vi "_readEscapeSequence.vi"(8 "error in (no error)":errorcluster, 11 "tJSONParser in":refnum<class "tJSONParser.lvclass">) -> (0 "error out":errorcluster, 2 "String Out":string, 3 "tJSONParser out":refnum<class "tJSONParser.lvclass">)   [LabVIEW 2013, in "JSON.lvlib" / "tJSONParser.lvclass"]
doc: "Reads and validates an escape sequence from a string. Valid escape sequences are \\\", \\/, \\\\, \\b, \\f, \\n, \\r, \\t, and \\u. If \\u is encountered, the immediately following unicode code is read and validated. An error is returned if an invalid escape sequence is encountered."
uses:
  tJSONParser.lvclass
  tJSONParser.lvclass/tJSONParser.ctl
  _error.ctl
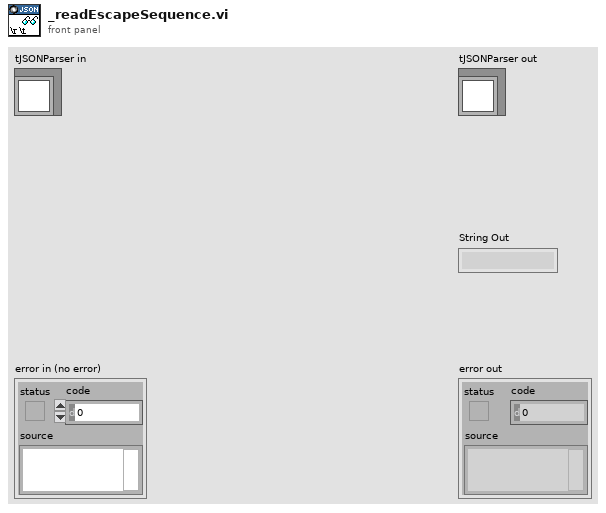
[diagram p1: front panel]
types:
  T1 = typedef "JSON.lvlib/tJSONParser.lvclass/_error.ctl" = enum16{"Missing Object Open", "Missing Pair Separator", "Missing Object End Or Separator", "Missing Pair String", "Unexpected Token", "Missing Array End Or Separator", "Invalid Escape Sequence", "Unexpected End Of File", "Invalid Unicode", "Unexpected End Of Line", "Invalid Numerical Constant"}
  T2 = typedef "JSON.lvlib/tJSONParser.lvclass/_tokenType.ctl" = enum16{"Object Begin", "Object End", "Array Begin", "Array End", "String Delimeter", "Forward Slash", "Number", "Boolean", "Null", "Object Or Array Separator", "Pair Separator", "End Of File", "Asterisk", "Backward Slash", "Other"}
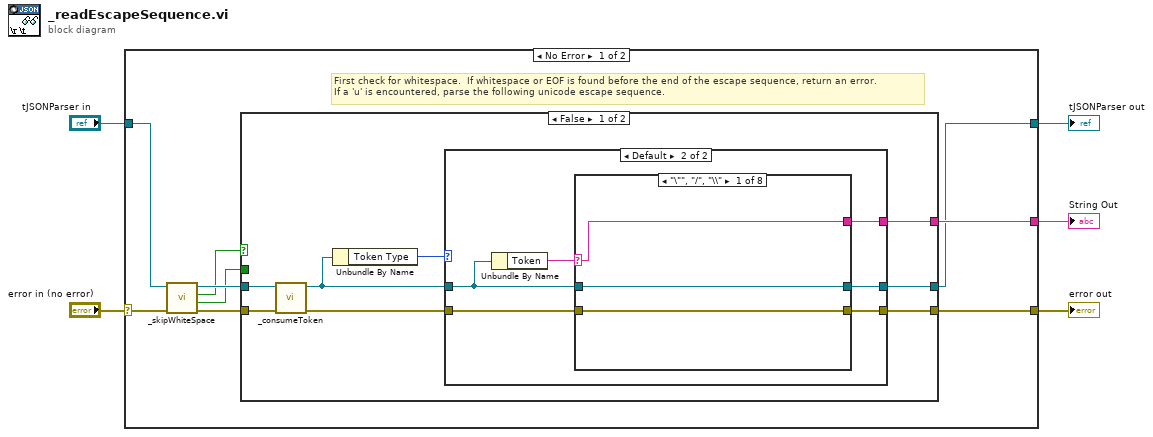
[diagram p0: block diagram]
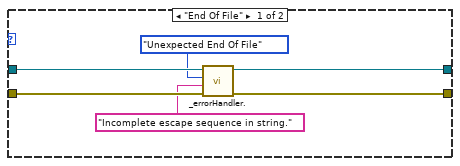
[diagram p2: hidden frame]
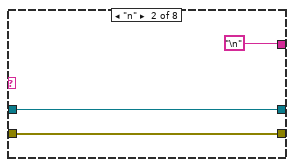
[diagram p3: hidden frame]
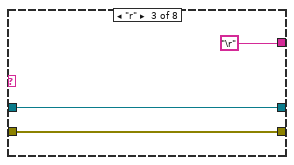
[diagram p4: hidden frame]
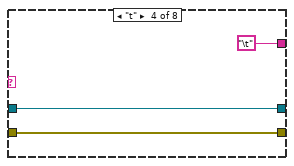
[diagram p5: hidden frame]
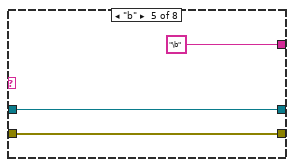
[diagram p6: hidden frame]
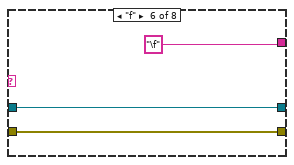
[diagram p7: hidden frame]
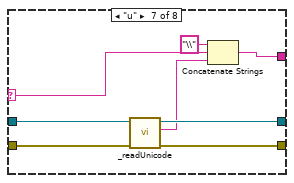
[diagram p8: hidden frame]
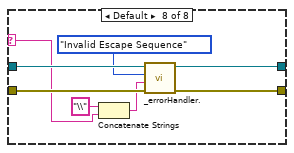
[diagram p9: hidden frame]
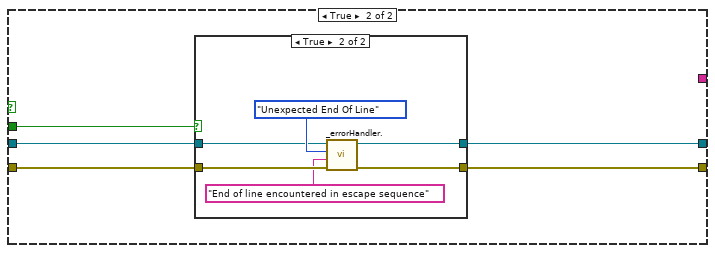
[diagram p10: hidden frame]
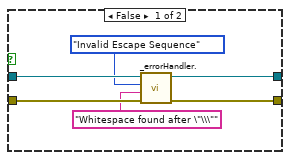
[diagram p11: hidden frame]
diagram:
  n1 = case shown="No Error" "error in (no error)" {
    selector: "error in (no error)" -> [w9 w87]
    tunnel: [w13 w87] -> w4
    tunnel: [w12 w86] -> w2
    tunnel: "tJSONParser in" -> [w11 w86]
    tunnel: [w14 _] -> w1
    frame No Error {
      # "First check for whitespace.  If whitespace or EOF is found before the end of the escape sequence, return an error.\nIf a 'u' is encountered, parse the following unicode escape sequence."
      n2 = call "_skipWhiteSpace.vi"("error in (no error)"=w9, "JSON Parser In"=w11) -> ("error out"=w8:errorcluster, "EOL Found?"=w6:bool, "White Space Found?"=w7:bool, "JSON Parser Out"=w10:refnum<class "tJSONParser.lvclass">)  [unwired: 5 in, 1 out]
      n3 = case shown="False" w7 {
        tunnel: [w21 _] -> w14
        tunnel: [w20 w70] -> w13
        tunnel: [w19 w69] -> w12
        tunnel: w10 -> [w18 w71]
        tunnel: w8 -> [w17 w72]
        tunnel: w6 -> [_ w73]
        frame False {
          n4 = call "_consumeToken.vi"("error in (no error)"=w17, "JSON Parser In"=w18) -> ("error out"=w22:errorcluster, "JSON Parser Out"=w16:refnum<class "tJSONParser.lvclass">)  [unwired: 8 in]
          n5 = Unbundle By Name(w16) -> ("Token Type"=w15:T2)
          n6 = case shown="Default" w15 {
            tunnel: w22 -> [w28 w34]
            tunnel: w16 -> [w25 w33]
            tunnel: [_ w31] -> w21
            tunnel: [w27 w30] -> w20
            tunnel: [w26 w29] -> w19
            frame "End Of File" {
              n7 = call "_errorHandler..vi"("error in (no error)"=w28, "Additional Text"="Incomplete escape sequence in string.", "Error Type"=_error."Unexpected End Of File", "JSON Parser In"=w25) -> ("error out"=w27:errorcluster, "JSON Parser Out"=w26:refnum<class "tJSONParser.lvclass">)  [unwired: 6 in]
            }
            frame Default {
              n8 = Unbundle By Name(w33) -> ("Token"=w32:string)
              n9 = case shown="\"\\\"\", \"/\", \"\\\\\"" w32 {
                selector: w32 -> [w35 _ _ _ _ _ w55 w61]
                tunnel: w34 -> [w37 w38 w41 w44 w47 w50 w60 w68]
                tunnel: w33 -> [w36 w39 w42 w45 w48 w51 w58 w66]
                tunnel: [w35 "\n" "\r" "\t" "\b" "\f" w56 _] -> w31
                tunnel: [w37 w38 w41 w44 w47 w50 w59 w67] -> w30
                tunnel: [w36 w39 w42 w45 w48 w51 w57 w65] -> w29
                frame "\"", "/", "\\" {
                }
                frame "n" {
                }
                frame "r" {
                }
                frame "t" {
                }
                frame "b" {
                }
                frame "f" {
                }
                frame "u" {
                  n10 = call "_readUnicode.vi"("error in (no error)"=w60, "tJSONParser in"=w58) -> ("error out"=w59:errorcluster, "String Out"=w54:string, "tJSONParser out"=w57:refnum<class "tJSONParser.lvclass">)  [unwired: 7 in]
                  n11 = Concatenate Strings("\\" ("string"), w55, w54) -> (w56:string)
                }
                frame Default {
                  n12 = Concatenate Strings("\\" ("string"), w61) -> (w63:string)
                  n13 = call "_errorHandler..vi"("error in (no error)"=w68, "Additional Text"=w63, "Error Type"=_error."Invalid Escape Sequence", "JSON Parser In"=w66) -> ("error out"=w67:errorcluster, "JSON Parser Out"=w65:refnum<class "tJSONParser.lvclass">)  [unwired: 6 in]
                }
              }
            }
          }
        }
        frame True {
          n14 = case shown="True" w73 {
            tunnel: w72 -> [w79 w85]
            tunnel: w71 -> [w77 w82]
            tunnel: [w78 w84] -> w70
            tunnel: [w76 w81] -> w69
            frame False {
              n15 = call "_errorHandler..vi"("error in (no error)"=w79, "Additional Text"="Whitespace found after \"\\\"", "Error Type"=_error."Invalid Escape Sequence", "JSON Parser In"=w77) -> ("error out"=w78:errorcluster, "JSON Parser Out"=w76:refnum<class "tJSONParser.lvclass">)  [unwired: 6 in]
            }
            frame True {
              n16 = call "_errorHandler..vi"("error in (no error)"=w85, "Additional Text"="End of line encountered in escape sequence", "Error Type"=_error."Unexpected End Of Line", "JSON Parser In"=w82) -> ("error out"=w84:errorcluster, "JSON Parser Out"=w81:refnum<class "tJSONParser.lvclass">)  [unwired: 6 in]
            }
          }
        }
      }
    }
    frame Error {
    }
  }
  "error out" <- w4
  "tJSONParser out" <- w2
  "String Out" <- w1
